vi "Perform_large_file_Analysis.vi"(7 "error in":errorcluster) -> (2 "Wvfm":waveform(dbl)[](array[waveform]), 3 "Filtered Nb of Events":i32, 5 "Total Nb of Events":dbl)   [LabVIEW 2019]
uses:
  <vilib>/Utility/error.llb/DialogType.ctl
  ESA_Data_Analysis_Global_VIs.vi
  SiPM_Tests_Global_Var.vi
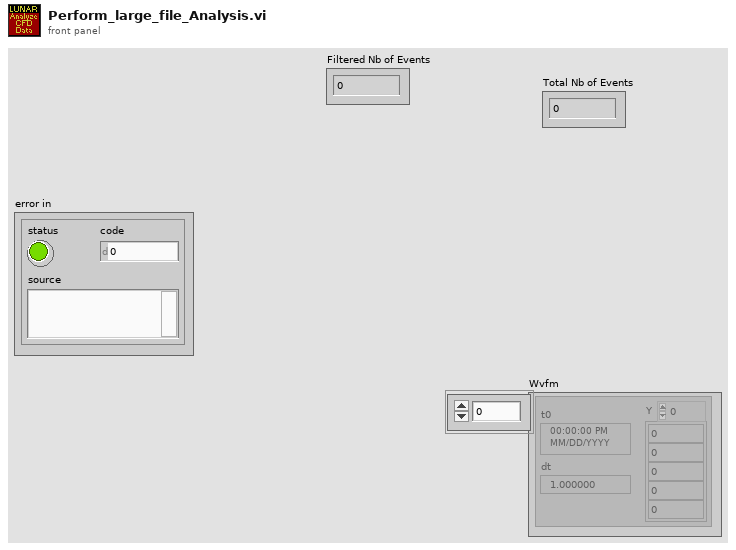
[diagram p1: front panel]
types:
  T1 = typedef "DialogType.ctl" = u16
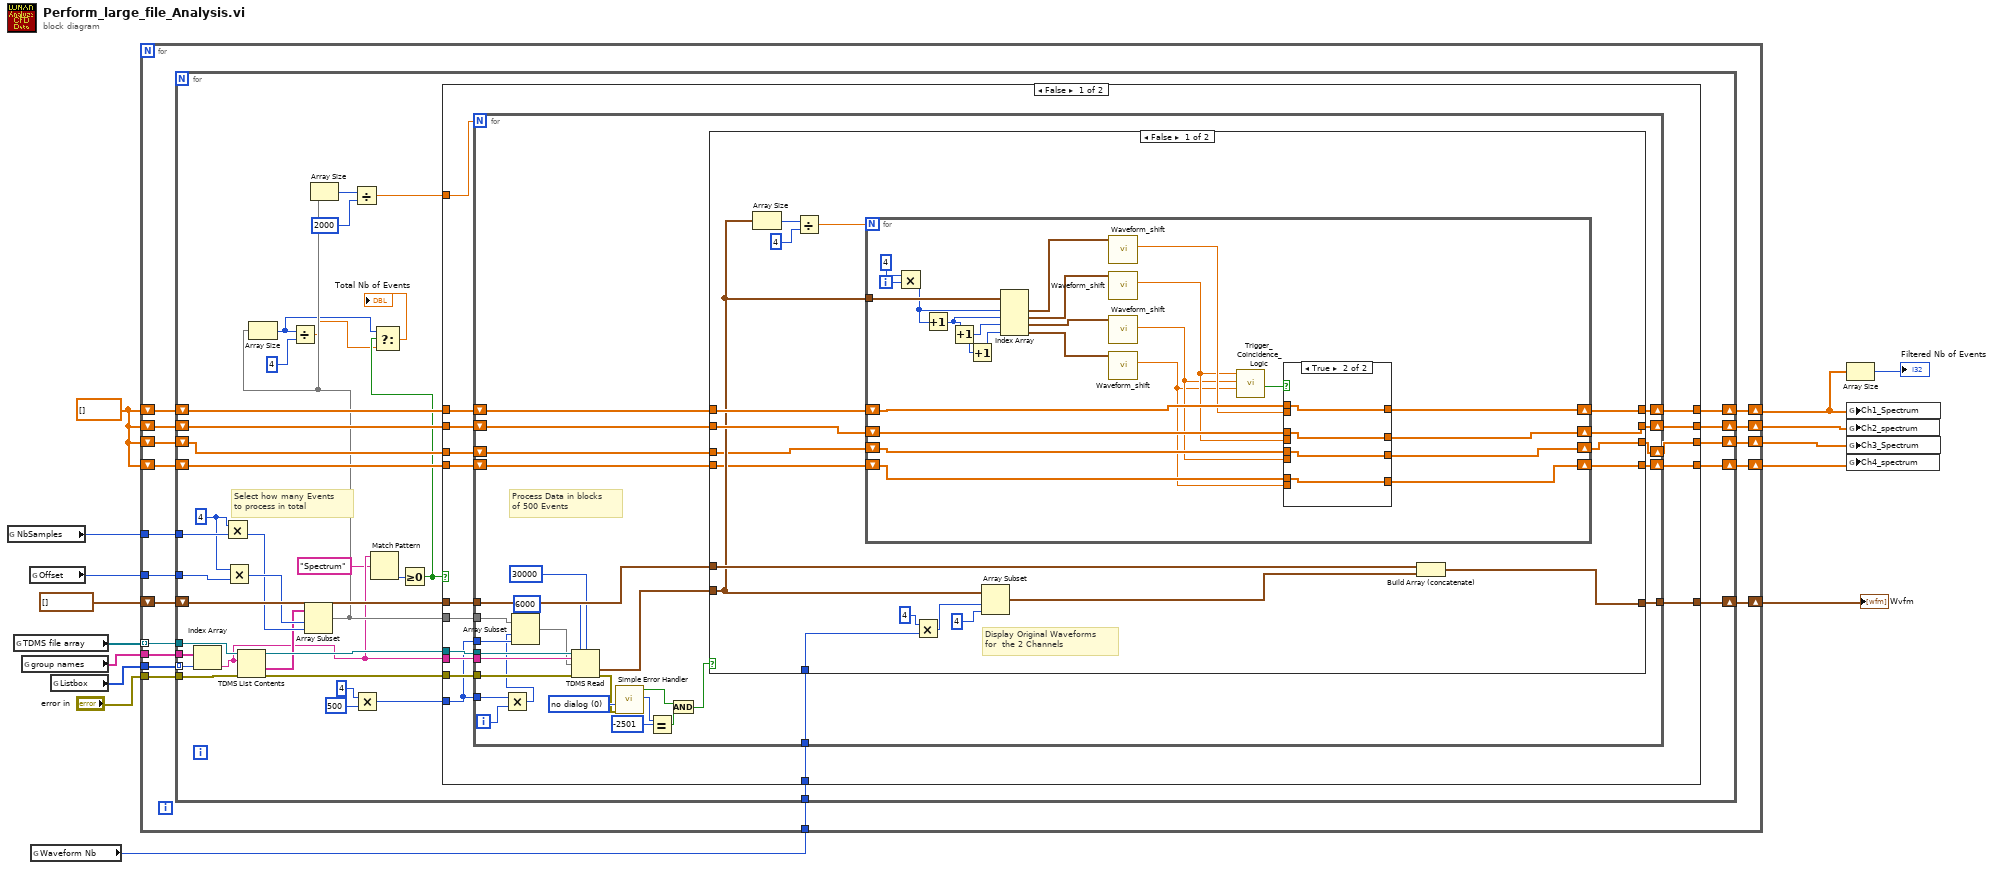
[diagram p0: block diagram]
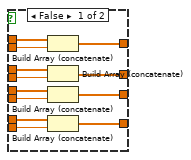
[diagram p2: hidden frame]
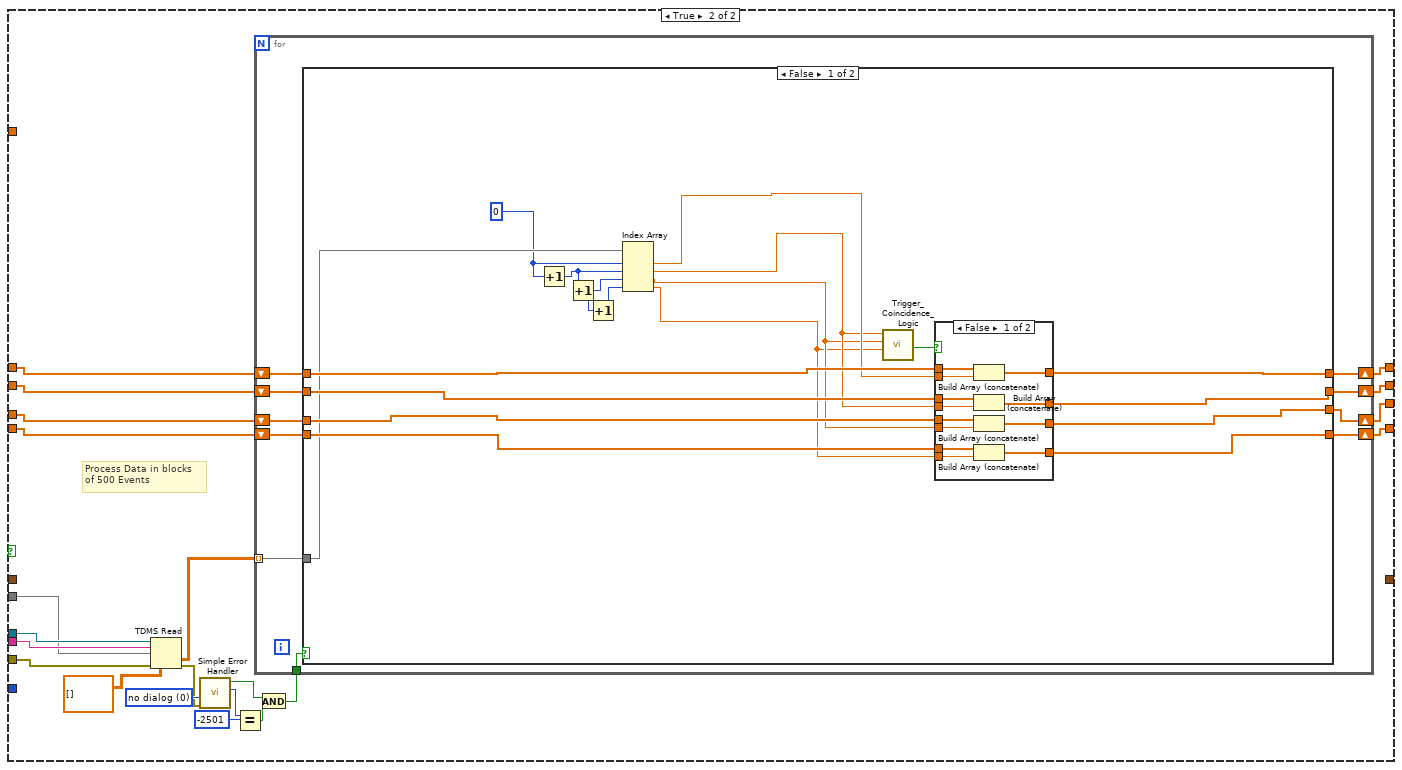
[diagram p4: hidden frame]
diagram:
  w5 = dbl[] []
  n1 = global read "SiPM_Tests_Global_Var.vi" "NbSamples"() -> (w8:i64)
  n2 = global read "SiPM_Tests_Global_Var.vi" "TDMS file array"() -> (w12:refnum<k34>[])
  n3 = global read "ESA_Data_Analysis_Global_VIs.vi" "group names"() -> (w15:string[])
  n4 = global read "SiPM_Tests_Global_Var.vi" "Offset"() -> (w10:i64)
  n5 = global read "SiPM_Tests_Global_Var.vi" "Waveform Nb"() -> (w7:u16)
  n6 = global read "ESA_Data_Analysis_Global_VIs.vi" "Listbox"() -> (w14:i32[])
  n7 = for {
    tunnel: w12 -> [w32] mode=indexing
    tunnel: w15 -> [w31]
    tunnel: w14 -> [w30]
    tunnel: "error in" -> [w29]
    tunnel: w10 -> [w27]
    shift-right: [w28] -> w11
    shift-left: waveform(dbl)[] [] -> [w26]
    shift-right: [w22] -> w6
    shift-left: w5 -> [w25]
    shift-right: [w23] -> w2
    shift-left: w5 -> [w24]
    tunnel: w8 -> [w21]
    tunnel: w7 -> [w20]
    shift-right: [w17] -> w4
    shift-left: w5 -> [w19]
    shift-right: [w16] -> w3
    shift-left: w5 -> [w18]
    n8 = for {
      tunnel: w32 -> [w70]
      tunnel: w31 -> [w69]
      tunnel: w30 -> [w68] mode=indexing
      tunnel: w29 -> [w67]
      tunnel: w27 -> [w57]
      shift-right: [w64] -> w28
      shift-left: w26 -> [w63]
      shift-right: [w59] -> w22
      shift-left: w25 -> [w62]
      shift-right: [w60] -> w23
      shift-left: w24 -> [w61]
      tunnel: w21 -> [w56]
      tunnel: w20 -> [w58]
      shift-right: [w52] -> w17
      shift-left: w19 -> [w54]
      shift-right: [w51] -> w16
      shift-left: w18 -> [w53]
      w55 = i64 4 ("x")
      # "Select how many Events \nto process in total"
      n9 = Index Array(array=w69, index=w68) -> (element=w39:string)
      n10 = Multiply(x=w55, y=w56) -> (x*y=w49:i64)
      n11 = Multiply(x=w55, y=w57) -> (x*y=w50:i64)
      n12 = TDMS List Contents(4:w67, 6:w39, 7:w70) -> (0:w65:errorcluster, 1:w48:string[], 3:w66:refnum<k34>)  [unwired: 1 out]
      n13 = Array Subset(array=w48, index=w50, length=w49) -> (w40:string[])
      n14 = Array Size(array=w40) -> (size(s)=w35:i32)
      n15 = Divide(x=w35, y=4) -> (x/y=w34:dbl)
      n16 = Array Size(array=w40) -> (size(s)=w43:i32)
      n17 = Divide(x=w43, y=2000) -> (x/y=w42:dbl)
      n18 = Multiply(x=i64 4, y=i64 500) -> (x*y=w45:i64)
      n19 = Match Pattern(string=w39, regular expression="Spectrum") -> (offset past match=w37:i32)  [unwired: 1 in, 3 out]
      n20 = Greater Or Equal To 0?(x=w37) -> (x >= 0?=w36:bool)
      n21 = Select(t=w35, s=w36, f=w34) -> (s? t:f=→"Total Nb of Events":dbl)
      n22 = case shown="False" w36 {
        tunnel: w66 -> [w87 w200]
        tunnel: w39 -> [w86 w201]
        tunnel: w65 -> [w85 w202]
        tunnel: [w84 _] -> w64
        tunnel: w63 -> [w83 _]
        tunnel: w62 -> [w82 w190]
        tunnel: w61 -> [w81 w191]
        tunnel: [w80 w187] -> w60
        tunnel: [w79 w186] -> w59
        tunnel: w58 -> [w78 _]
        tunnel: w54 -> [w77 w189]
        tunnel: w53 -> [w76 w188]
        tunnel: [w75 w185] -> w52
        tunnel: [w74 w184] -> w51
        tunnel: w45 -> [w73 _]
        tunnel: w42 -> [w72 _]
        tunnel: w40 -> [w71 w183]
        frame False {
          n23 = for {
            N: w72 -> [_]
            tunnel: w87 -> [w117]
            tunnel: w86 -> [w116]
            tunnel: w85 -> [w113]
            tunnel: [w112] -> w84
            tunnel: w83 -> [w111]
            tunnel: w78 -> [w101]
            tunnel: w71 -> [w95]
            shift-right: [w103] -> w80
            shift-left: w81 -> [w104]
            shift-right: [w102] -> w79
            shift-left: w82 -> [w105]
            shift-right: [w98] -> w75
            shift-left: w77 -> [w100]
            shift-right: [w97] -> w74
            shift-left: w76 -> [w99]
            tunnel: w73 -> [w93]
            tunnel: w73 -> [w91]
            i -> [w92]
            w115 = T1 0 items=["no dialog", "OK message", "continue or stop message", "OK message + warnings", "continue/stop + warnings"] ("type of dialog (OK msg:1)")
            # "Process Data in blocks \nof 500 Events"
            n24 = Multiply(x=w91, y=w92) -> (x*y=w90:i64)
            n25 = Array Subset(array=w95, index=w90, length=w93) -> (w94:string[])
            n26 = TDMS Read(0:w117, 1:i64 6000 ("offset (0)"), 2:i64 30000 ("count (-1: all)"), 5:w116, 7:w94, 11:w113) -> (10:w96:waveform(dbl)[], 15:w114:errorcluster)  [unwired: 2 in, 4 out]
            n27 = call <vilib>:"Simple Error Handler.vi"("type of dialog (OK msg:1)"=w115, "error in (no error)"=w114) -> ("error?"=w109:bool, "code out"=w108:i32)  [unwired: 3 in, 3 out]
            n28 = Equal?(x=w108, y=-2501) -> (x = y?=w106:bool)
            n29 = And(x=w109, y=w106) -> (x .and. y?=w110:bool)
            n30 = case shown="False" w110 {
              tunnel: w96 -> [w122 _]
              tunnel: [w135 w181] -> w112
              tunnel: w111 -> [w134 w181]
              tunnel: w105 -> [w130 w179]
              tunnel: w104 -> [w129 w180]
              tunnel: [w128 w180] -> w103
              tunnel: [w127 w179] -> w102
              tunnel: w101 -> [w123 _]
              tunnel: w100 -> [w121 w178]
              tunnel: w99 -> [w120 w177]
              tunnel: [w119 w178] -> w98
              tunnel: [w118 w177] -> w97
              frame False {
                # "Display Original Waveforms\nfor  the 2 Channels"
                n31 = Array Size(array=w122) -> (size(s)=w133:i32)
                n32 = Divide(x=w133, y=4) -> (x/y=w131:dbl)
                n33 = for {
                  N: w131 -> [_]
                  tunnel: w122 -> [w160]
                  shift-right: [w147] -> w128
                  shift-left: w129 -> [w148]
                  shift-right: [w145] -> w127
                  shift-left: w130 -> [w155]
                  shift-right: [w143] -> w119
                  shift-left: w121 -> [w144]
                  shift-right: [w142] -> w118
                  shift-left: w120 -> [w141]
                  i -> [w154]
                  n34 = Multiply(x=4, y=w154) -> (x*y=w158:i32)
                  n35 = Increment(x=w158) -> (x+1=w153:i32)
                  n36 = Increment(x=w153) -> (x+1=w151:i32)
                  n37 = Increment(x=w151) -> (x+1=w152:i32)
                  n38 = Index Array(array=w160, index #1=w158, index #2=w153, index #3=w151, index #4=w152) -> (element #1=w157:waveform(dbl), element #2=w156:waveform(dbl), element #3=w150:waveform(dbl), element #4=w149:waveform(dbl))
                  n39 = call "Waveform_shift.vi"("Waveform_in"=w157) -> ("Peak Value"=w146:dbl)  [unwired: 9 in]
                  n40 = call "Waveform_shift.vi"("Waveform_in"=w156) -> ("Peak Value"=w139:dbl)  [unwired: 9 in]
                  n41 = call "Waveform_shift.vi"("Waveform_in"=w150) -> ("Peak Value"=w138:dbl)  [unwired: 9 in]
                  n42 = call "Waveform_shift.vi"("Waveform_in"=w149) -> ("Peak Value"=w137:dbl)  [unwired: 9 in]
                  n43 = call "Trigger_Coincidence_Logic.vi"("Peak_ch4"=w137, "Peak_ch3"=w138, "Peak_ch2"=w139) -> ("Filter-out"=w140:bool)  [unwired: 8 in]
                  n44 = case shown="True" w140 {
                    tunnel: w155 -> [w172 w175]
                    tunnel: w139 -> [w171 _]
                    tunnel: w148 -> [w170 w176]
                    tunnel: [w169 w176] -> w147
                    tunnel: w146 -> [w168 _]
                    tunnel: [w167 w175] -> w145
                    tunnel: w144 -> [w166 w174]
                    tunnel: w138 -> [w165 _]
                    tunnel: [w164 w174] -> w143
                    tunnel: [w163 w173] -> w142
                    tunnel: w141 -> [w162 w173]
                    tunnel: w137 -> [w161 _]
                    frame False {
                      n45 = Build Array (concatenate)(w170, w168) -> (w169:dbl[])
                      n46 = Build Array (concatenate)(w172, w171) -> (w167:dbl[])
                      n47 = Build Array (concatenate)(w166, w165) -> (w164:dbl[])
                      n48 = Build Array (concatenate)(w162, w161) -> (w163:dbl[])
                    }
                    frame True {
                    }
                  }
                }
                n49 = Multiply(x=4, y=w123) -> (x*y=w126:i32)
                n50 = Array Subset(array=w122, index=w126, length=4) -> (w136:waveform(dbl)[])
                n51 = Build Array (concatenate)(w134, w136) -> (w135:waveform(dbl)[])
              }
              frame True {
              }
            }
          }
        }
        frame True {
          w199 = T1 0 items=["no dialog", "OK message", "continue or stop message", "OK message + warnings", "continue/stop + warnings"] ("type of dialog (OK msg:1)")
          # "Process Data in blocks \nof 500 Events"
          n52 = TDMS Read(0:w200, 5:w201, 7:w183, 11:w202, 12:dbl[][] []) -> (10:w192:dbl[][], 15:w198:errorcluster)  [unwired: 3 in, 4 out]
          n53 = call <vilib>:"Simple Error Handler.vi"("type of dialog (OK msg:1)"=w199, "error in (no error)"=w198) -> ("error?"=w196:bool, "code out"=w195:i32)  [unwired: 3 in, 3 out]
          n54 = Equal?(x=w195, y=-2501) -> (x = y?=w193:bool)
          n55 = And(x=w196, y=w193) -> (x .and. y?=w197:bool)
          n56 = for {
            tunnel: w197 -> [w212]
            tunnel: w192 -> [w211] mode=indexing
            shift-right: [w203] -> w184
            shift-left: w188 -> [w207]
            shift-right: [w204] -> w185
            shift-left: w189 -> [w208]
            shift-right: [w205] -> w186
            shift-left: w190 -> [w209]
            shift-right: [w206] -> w187
            shift-left: w191 -> [w210]
            n57 = case shown="False" w212 {
              tunnel: w209 -> [w230 w249]
              tunnel: w210 -> [w229 w250]
              tunnel: [w228 w250] -> w206
              tunnel: [w227 w249] -> w205
              tunnel: w208 -> [w226 w248]
              tunnel: w207 -> [w225 w247]
              tunnel: [w224 w248] -> w204
              tunnel: [w223 w247] -> w203
              tunnel: w211 -> [w222 _]
              frame False {
                w213 = 0 ("x")
                n58 = Increment(x=w213) -> (x+1=w221:i32)
                n59 = Increment(x=w221) -> (x+1=w219:i32)
                n60 = Increment(x=w219) -> (x+1=w220:i32)
                n61 = Index Array(array=w222, index #1=w213, index #2=w221, index #3=w219, index #4=w220) -> (element #1=w217:dbl, element #2=w216:dbl, element #3=w215:dbl, element #4=w214:dbl)
                n62 = call "Trigger_Coincidence_Logic.vi"("Peak_ch4"=w214, "Peak_ch3"=w215, "Peak_ch2"=w216) -> ("Filter-out"=w218:bool)  [unwired: 8 in]
                n63 = case shown="False" w218 {
                  tunnel: w230 -> [w242 w245]
                  tunnel: w216 -> [w241 _]
                  tunnel: w229 -> [w240 w246]
                  tunnel: [w239 w246] -> w228
                  tunnel: w217 -> [w238 _]
                  tunnel: [w237 w245] -> w227
                  tunnel: w226 -> [w236 w244]
                  tunnel: w215 -> [w235 _]
                  tunnel: [w234 w244] -> w224
                  tunnel: [w233 w243] -> w223
                  tunnel: w225 -> [w232 w243]
                  tunnel: w214 -> [w231 _]
                  frame False {
                    n64 = Build Array (concatenate)(w240, w238) -> (w239:dbl[])
                    n65 = Build Array (concatenate)(w242, w241) -> (w237:dbl[])
                    n66 = Build Array (concatenate)(w236, w235) -> (w234:dbl[])
                    n67 = Build Array (concatenate)(w232, w231) -> (w233:dbl[])
                  }
                  frame True {
                  }
                }
              }
              frame True {
              }
            }
          }
        }
      }
    }
  }
  "Wvfm" <- w11
  n68 = Array Size(array=w2) -> (size(s)=→"Filtered Nb of Events":i32)
  n69 = global write "SiPM_Tests_Global_Var.vi" "Ch1_Spectrum"(w2) -> ()
  n70 = global write "SiPM_Tests_Global_Var.vi" "Ch2_spectrum"(w6) -> ()
  n71 = global write "SiPM_Tests_Global_Var.vi" "Ch3_Spectrum"(w4) -> ()
  n72 = global write "SiPM_Tests_Global_Var.vi" "Ch4_spectrum"(w3) -> ()
